vi "Flip Flop.vi"(9 "Line 2":bool, 10 "Line 1":bool) -> (2 "Switch":bool)   [LabVIEW 2018]
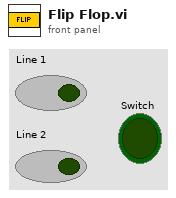
[diagram p1: front panel]
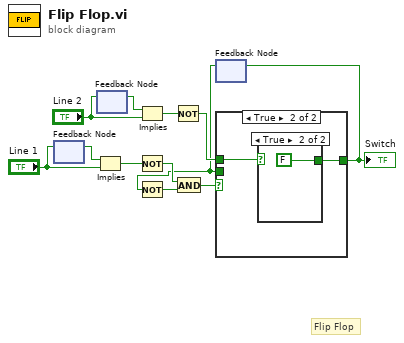
[diagram p0: block diagram]
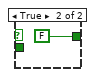
[diagram p3: hidden frame]
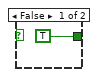
[diagram p4: hidden frame]
diagram:
  # "Flip Flop"
  n1 = feedback #1() -> (w4:bool)  [unwired: 1 in]
  n2 = feedback-in #1("Line 1") -> ()
  n3 = Implies(1:"Line 1", 2:w4) -> (0:w12:bool)
  n4 = feedback #2() -> (w2:bool)  [unwired: 1 in]
  n5 = feedback-in #2("Line 2") -> ()
  n6 = Implies(1:"Line 2", 2:w2) -> (0:w8:bool)
  n7 = Not(x=w12) -> (.not. x?=w10:bool)
  n8 = Not(x=w8) -> (.not. x?=w7:bool)
  n9 = feedback #3() -> (w5:bool)  [unwired: 1 in]
  n10 = Not(x=w5) -> (.not. x?=w11:bool)
  n11 = And(x=w10, y=w11) -> (x .and. y?=w9:bool)
  n12 = case shown="True" w9 {
    tunnel: w7 -> [w15 w19]
    tunnel: [w14 w18] -> w6
    tunnel: w5 -> [w13 _]
    frame False {
      n13 = case shown="False" w15 {
        tunnel: [w16 FALSE] -> w14
        tunnel: w13 -> [w16 _]
        frame False {
        }
        frame True {
        }
      }
    }
    frame True {
      n14 = case shown="True" w19 {
        tunnel: [TRUE FALSE] -> w18
        frame False {
        }
        frame True {
        }
      }
    }
  }
  "Switch" <- w6
  n15 = feedback-in #3(w6) -> ()
